vi "For主程序.vi"() -> ()   [LabVIEW 2016]
panel:
  in  "输入n计算阶乘":dbl
  out "阶乘为":dbl
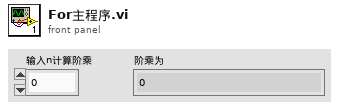
[diagram p1: front panel]
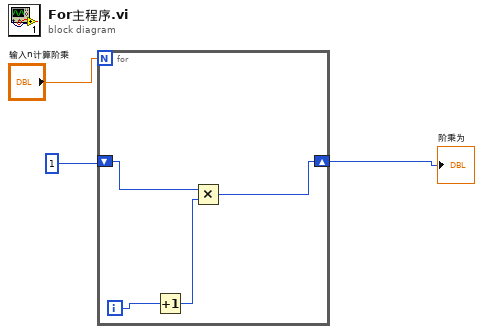
[diagram p0: block diagram]
diagram:
  n1 = for {
    N: "输入n计算阶乘" -> [_]
    shift-right: [w4] -> w1
    shift-left: 1 -> [w6]
    i -> [w7]
    n2 = Increment(x=w7) -> (x+1=w5:i32)
    n3 = Multiply(x=w6, y=w5) -> (x*y=w4:i32)
  }
  "阶乘为" <- w1
